vi "系统设置.vi"() -> ()   [LabVIEW 2016]
uses:
  <vilib>/Utility/miscctls.llb/LVPointTypeDef.ctl
  <vilib>/ptbypt/NI_PtbyPt.lvlib
  <vilib>/Utility/config.llb/NI_LVConfig.lvlib
  PLC/PLC.lvlib
panel:
  in  "模块启用配置":bool
  in  "短信报警设置":bool
  in  "首页显示设置":bool
  in  "跨度核查":bool
  in  "空白核查":bool
  out "选项卡控件":enum32{"自由设定", "国标协议", "流量设定"}(tab)
  in  "24H周期设置":bool[](xcontrol)
  in  "运行间隔":i16=4 min=1 max=24
  in  "流量阈值":dbl=4.0 min=1.0 max=24.0
  in  "时间阈值":u16=4 min=1 max=24
  in  "周期设置":enum16{"自由设定", "国标协议", "流量设定"}(ring)
  out "x = y?":bool
  in  "质控启动日期":string(combo)="关闭"
  in  "跨度核查时间":u16(ring)=6 items=["00H", "01H", "02H", "03H", "04H", "05H", "06H", "07H", "08H", "09H", "10H", "11H", "12H", "13H", "14H", "15H", "16H", "17H", "18H", "19H", "20H", "21H", "22H", "23H", "关闭"]
  in  "空白核查时间":u16(ring)=2 items=["00H", "01H", "02H", "03H", "04H", "05H", "06H", "07H", "08H", "09H", "10H", "11H", "12H", "13H", "14H", "15H", "16H", "17H", "18H", "19H", "20H", "21H", "22H", "23H", "关闭"]
  in  "CODCr":bool
  in  "总磷总氮":bool
  in  "氨氮":bool
  in  "CODmn":bool
  in  "多参数":bool
  in  "输入密码":dbl
  in  "布尔":bool
  in  "副屏显示设置":bool
  in  "开机启动":bool caption="氨氮禁用"
  in  "运行模式":enum16{"维护模式", "常规模式", "应急模式", "质控模式"}(ring)
  # "注：周期设置分为自由设定和国标协议两种。\n1：选择自由设定情况下：运行间隔将不可选用并变灰色，周期设置可自由手动勾选\n2：选择国标协议情况下：周期时间将由运行间隔选择的时间决定，下方周期设置被禁用并无法手动勾选。\n3：选择流量设定情况下：瞬时流量连续超过流量阈值到达时间阈值设定值，仪器将自动开启测量。"
  # "自动运行启动参数"
  # "质控频次："
  # "空白核查时间："
  # "跨度核查时间："
  # "启动周期设置"
  # "m3/S"
  # "秒"
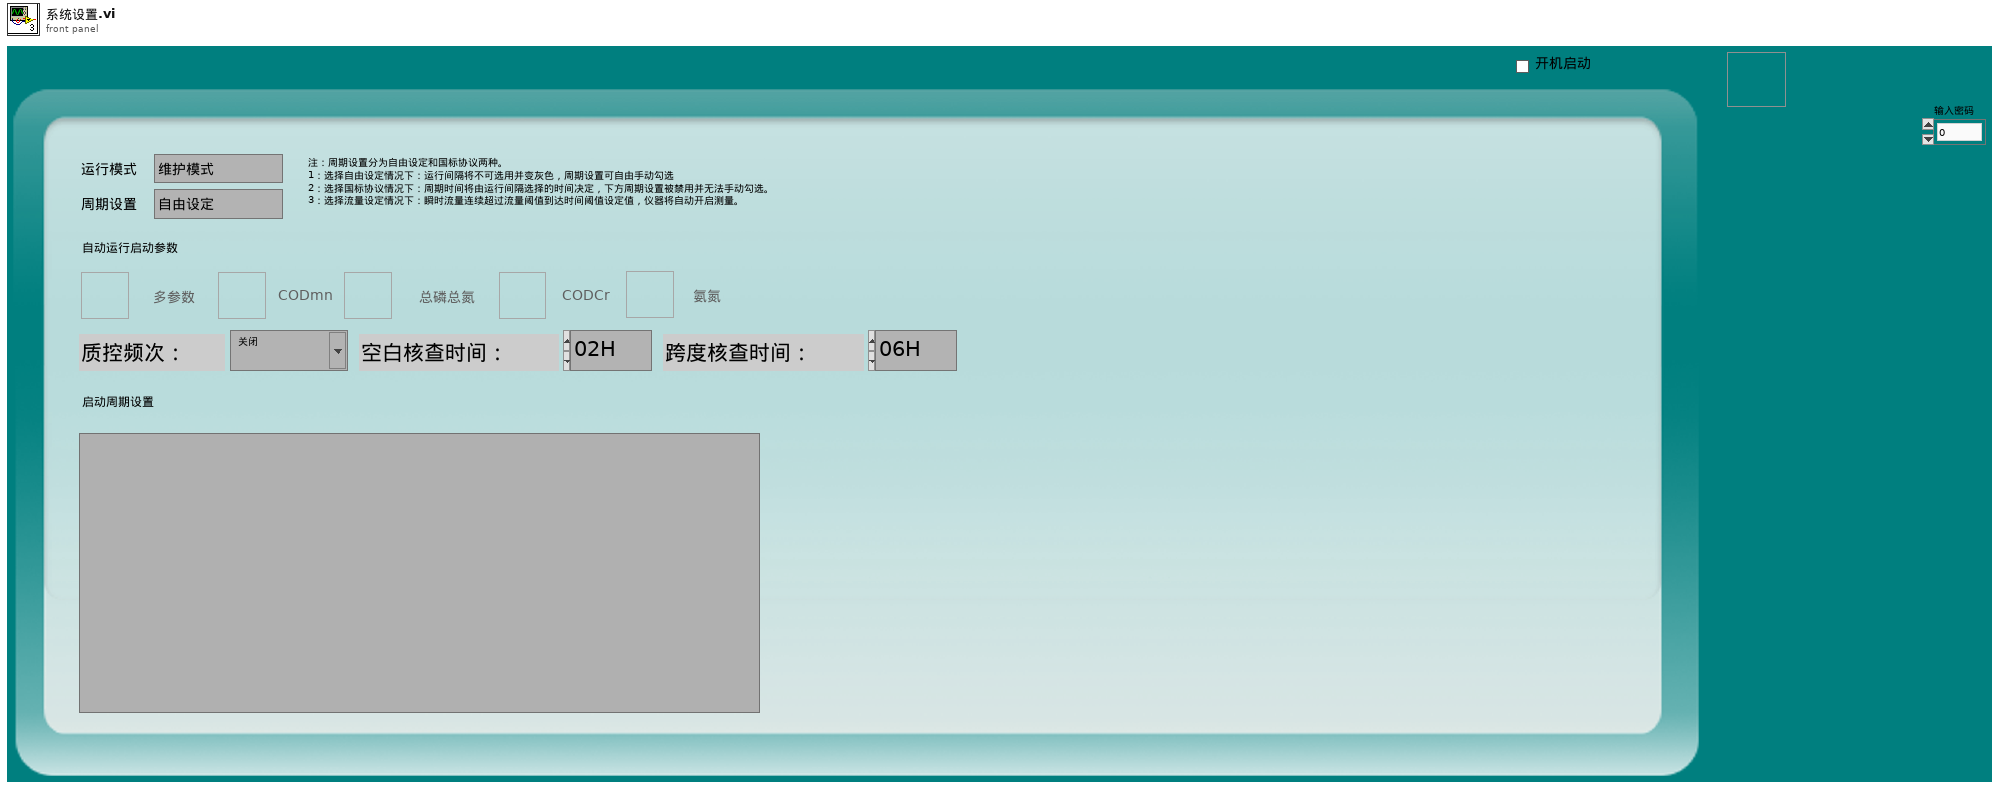
[diagram p1: front panel]
types:
  T1 = typedef "NI_LVConfig.lvlib/Config Data RefNum.ctl" = refnum<k1>
  T2 = typedef "LVPointTypeDef.ctl" = cluster{"Horizontal":i16, "Vertical":i16}
  T3 = enum8{"Enabled", "Disabled", "Disabled and Grayed Out"}
  T4 = enum32{"Bad", "Idle", "Run top level", "Running"}
  T5 = enum32{"Invalid", "Standard", "Closed", "Hidden", "Minimized", "Maximized"}
  T6 = cluster{"运行模式":enum16{"维护模式", "常规模式", "应急模式", "质控模式"}}
  T7 = cluster{"测量模式":enum16{"水样测量", "标样核查", "零点核查", "跨度核查", "空白测试", "加标回收", "平行样", "校零", "校标"}}
  T8 = cluster{"站号":u16, "量程切换":enum32{"H", "L", "AUTO"}, "控制命令":enum16{"启动测量", "标样核查", "零点核查", "跨度核查", "空白测试", "平行样测试", "加标回收", "空白校准", "标样校准", "初始化（清洗）", "停止测试", "仪器重启", "校时", "模式设置", "测量间隔设置"}, "模式设置":enum16{"待机", "连续模式", "周期模式", "定点模式", "受控模式", "手动模式"}, "测量间隔":u16}
  T9 = enum16{"启动测量", "标样核查", "零点核查", "跨度核查", "空白测试", "平行样测试", "加标回收", "空白校准", "标样校准", "初始化（清洗）", "停止测试", "仪器重启", "校时", "模式设置", "测量间隔设置"}
  T10 = cluster{"测试模式":enum16{"正常测试", "集成干预"}, "参数启用":cluster{"氨氮":bool, "总磷总氮":bool, "CODMn":bool, "CODcr":bool, "多参数":bool}}
  T11 = typedef "LVDateTimeRec.ctl" = cluster{"秒数的小数部分":dbl, "秒":i32, "分":i32, "时":i32, "日":i32, "月":i32, "年":i32, "天数（周）":i32, "天数（年）":i32, "DST":i32}
  T12 = cluster{"运行模式":enum16{"维护模式", "常规模式", "应急模式", "质控模式"}, "质控频次":enum16{"关闭", "每天", "星期一", "星期二", "星期三", "星期四", "星期五", "星期六", "星期日"}, "空白核查时间":u16, "跨度核查时间":u16, "24H周期设置":bool[]}
  T13 = cluster{"水样测试量程模式":enum16{"H", "L", "AUTO"}, "空白核查量程模式":enum16{"H", "L", "AUTO"}, "跨度核查量程模式":enum16{"H", "L", "AUTO"}}
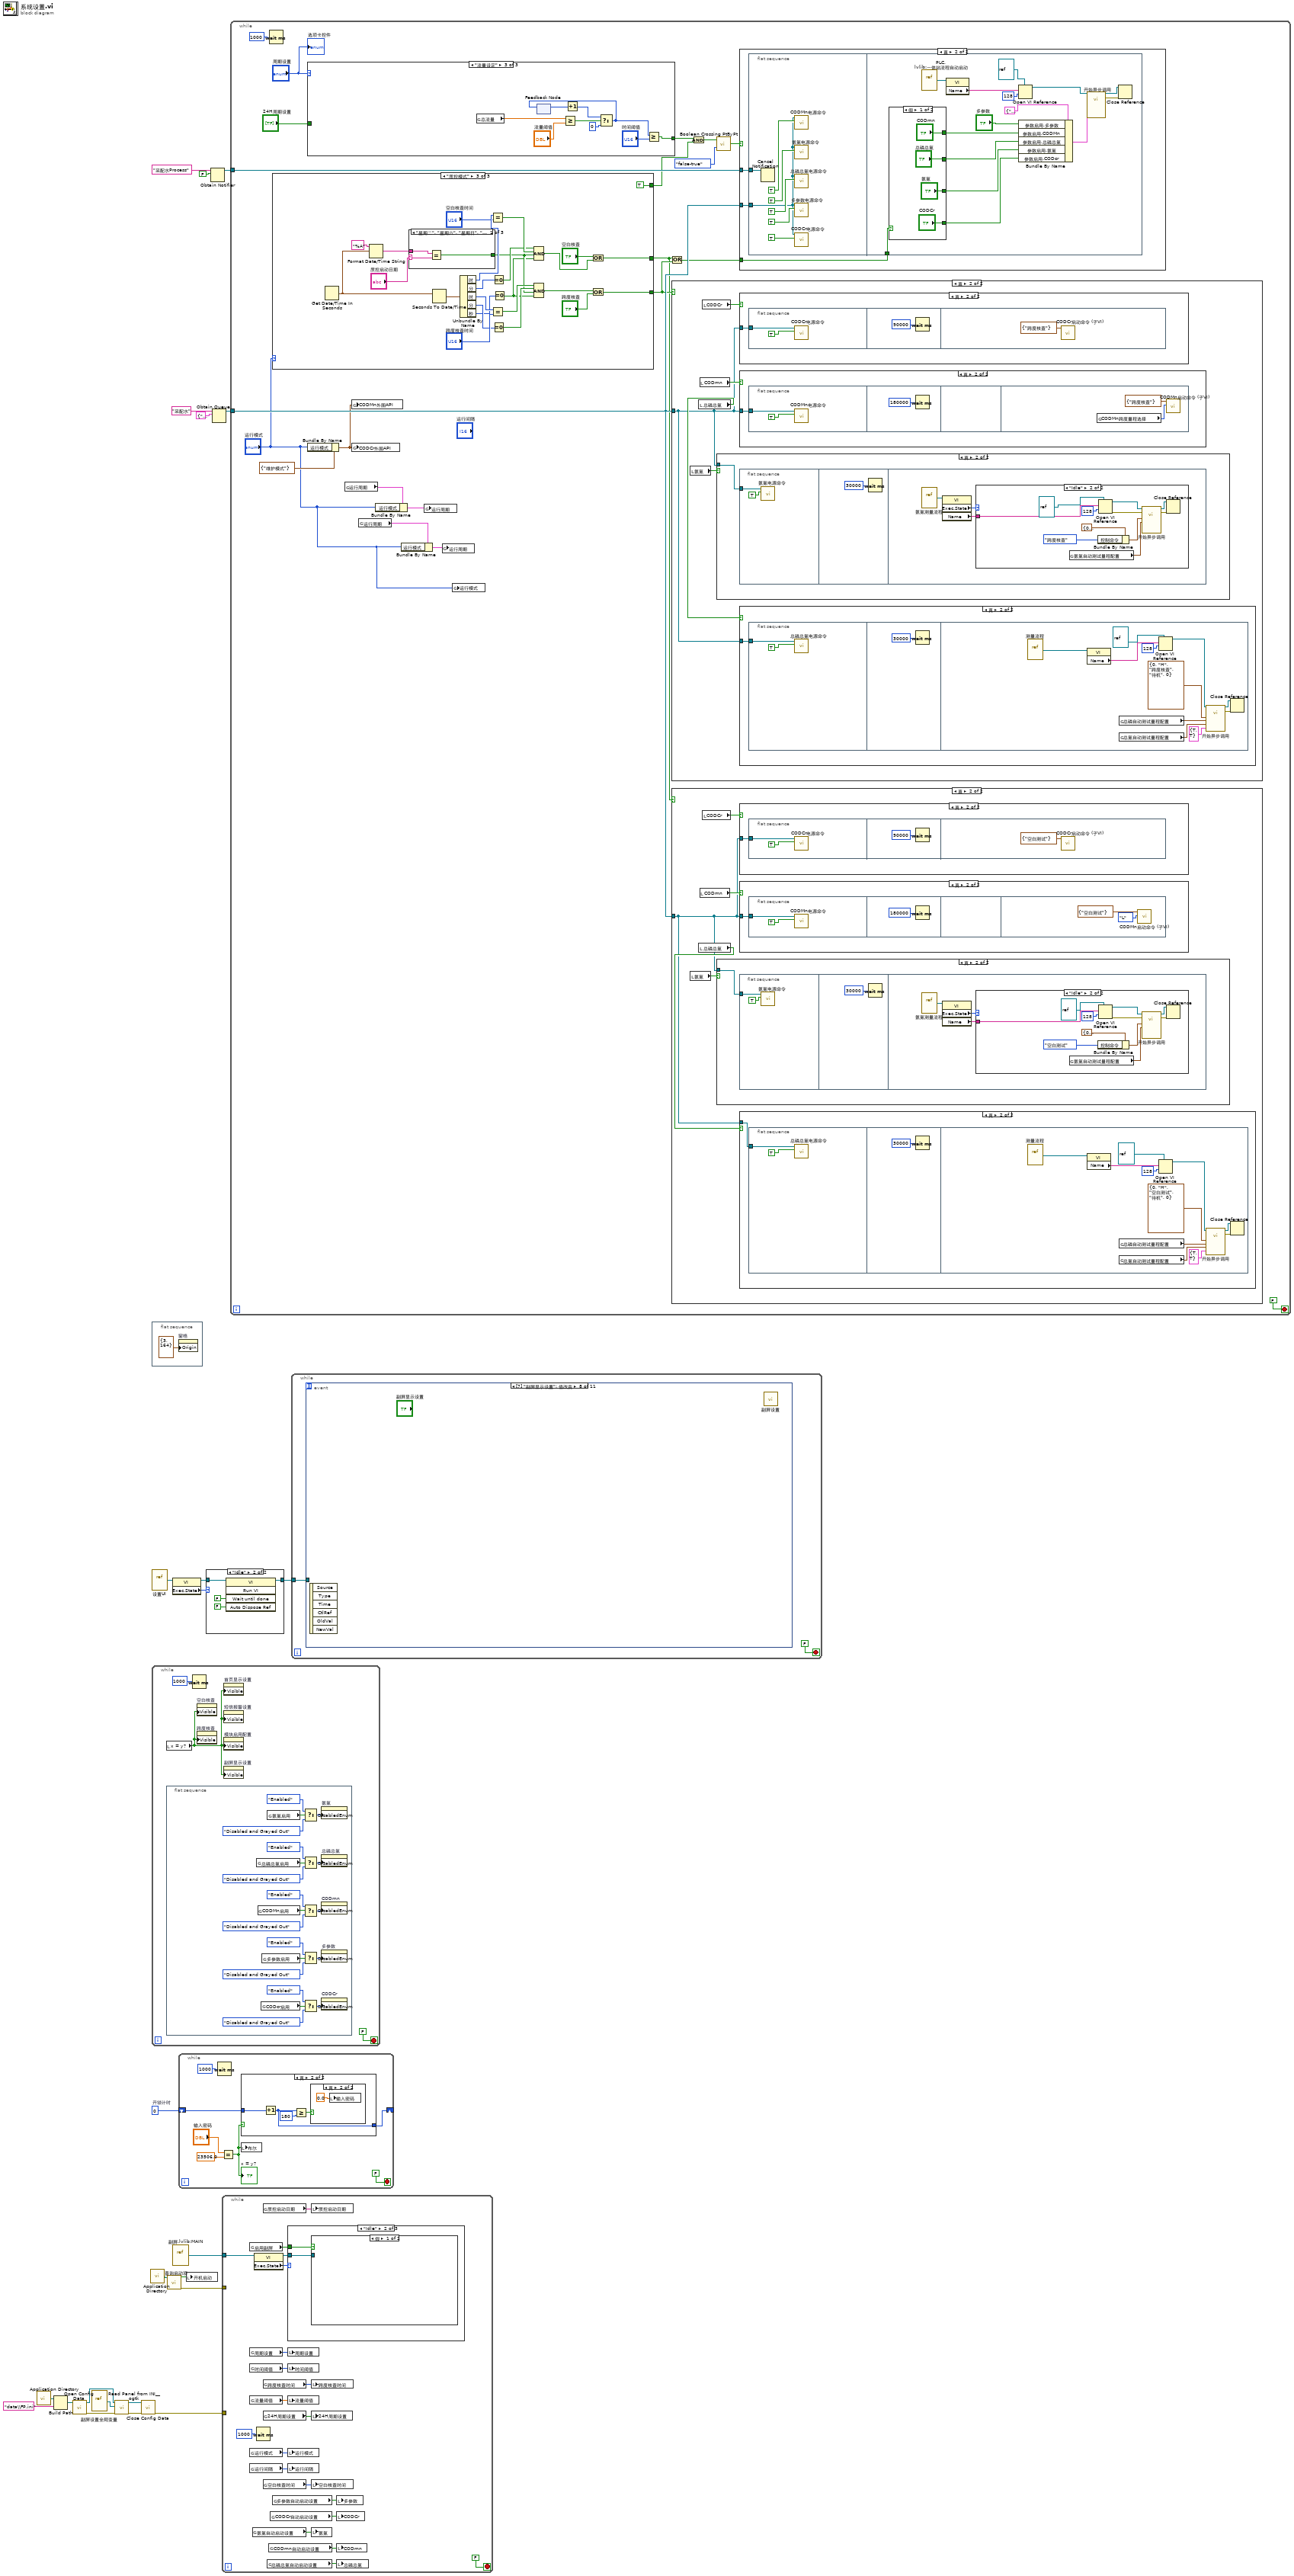
[diagram p0: block diagram]
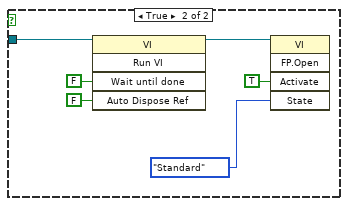
[diagram p6: hidden frame]
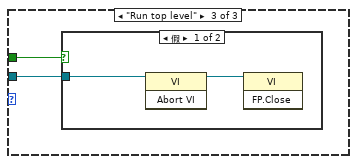
[diagram p7: hidden frame]
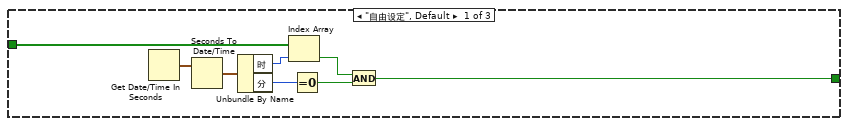
[diagram p9: hidden frame]
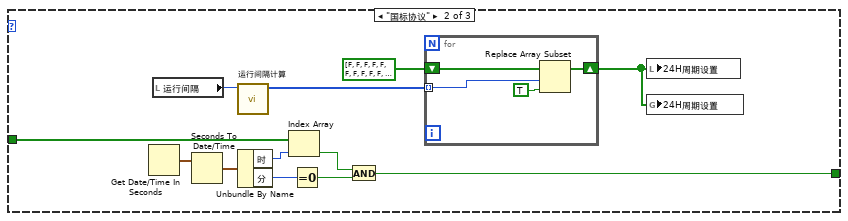
[diagram p10: hidden frame]
diagram:
  w19 = u32 0  # 开锁计时
  n1 = call <vilib>:"Application Directory.vi"() -> ("Application Directory"=w1:path)
  n2 = Build Path(base path=w1, name or relative path="data\\FP.ini" ("名称或相对路径")) -> (appended path=w8:path)
  n3 = call <vilib>:"Open Config Data.vi"("configuration file path"=w8) -> ("error out"=w7:errorcluster, "refnum"=w4:T1)  [unwired: 8 in, 1 out]
  n4 = vi-ref "副屏设置全局变量.vi"() -> (w5:refnum<vi>)
  n5 = call <userlib>:"Read Panel from INI__ogtk.vi"("error in (no error)"=w7, "VI ref"=w5, "refnum"=w4) -> ("error out"=w6:errorcluster, "refnum out"=w3:T1)  [unwired: 7 in]
  n6 = call <vilib>:"Close Config Data.vi"("error in (no error)"=w6, "refnum"=w3) -> ("error out"=w2:errorcluster)  [unwired: 8 in, 1 out]
  n7 = call <vilib>:"Application Directory.vi"() -> ("Application Directory"=w21:path)
  n8 = flat-sequence {
    frame #0 {
      n9 = property on="窗格" class="Pane"("Origin"=T2 {"Horizontal"=3, "Vertical"=164} ("原点")) -> ()  [unwired: 2 in, 2 out]
    }
  }
  n10 = vi-ref "设置UI.vi"() -> (w14:refnum<vi>)
  n11 = while {
    stop <- FALSE stop-if-true
    n12 = local read "x = y?"() -> (w26:bool)
    n13 = flat-sequence {
      frame #0 {
        n14 = global read "系统设置全局变量.vi" "总磷总氮启用"() -> (w36:bool)
        n15 = global read "系统设置全局变量.vi" "CODMn启用"() -> (w34:bool)
        n16 = global read "系统设置全局变量.vi" "CODcr启用"() -> (w35:bool)
        n17 = global read "系统设置全局变量.vi" "多参数启用"() -> (w33:bool)
        n18 = global read "系统设置全局变量.vi" "氨氮启用"() -> (w29:bool)
        n19 = Select(t=T3."Enabled" ("禁用"), s=w29, f=T3."Disabled and Grayed Out" ("禁用")) -> (s? t:f=w37:T3)
        n20 = Select(t=T3."Enabled" ("禁用"), s=w36, f=T3."Disabled and Grayed Out" ("禁用")) -> (s? t:f=w31:T3)
        n21 = Select(t=T3."Enabled" ("禁用"), s=w34, f=T3."Disabled and Grayed Out" ("禁用")) -> (s? t:f=w38:T3)
        n22 = Select(t=T3."Enabled" ("禁用"), s=w33, f=T3."Disabled and Grayed Out" ("禁用")) -> (s? t:f=w32:T3)
        n23 = Select(t=T3."Enabled" ("禁用"), s=w35, f=T3."Disabled and Grayed Out" ("禁用")) -> (s? t:f=w48:T3)
        n24 = property on="氨氮" class="Bool (严格)"("DisabledEnum"=w37) -> ()  [unwired: 2 in, 2 out]
        n25 = property on="总磷总氮" class="Bool (严格)"("DisabledEnum"=w31) -> ()  [unwired: 2 in, 2 out]
        n26 = property on="CODmn" class="Bool (严格)"("DisabledEnum"=w38) -> ()  [unwired: 2 in, 2 out]
        n27 = property on="多参数" class="Bool (严格)"("DisabledEnum"=w32) -> ()  [unwired: 2 in, 2 out]
        n28 = property on="CODCr" class="Bool (严格)"("DisabledEnum"=w48) -> ()  [unwired: 2 in, 2 out]
      }
    }
    n29 = Wait (ms)(milliseconds to wait=u32 1000 ("等待时间（毫秒）")) -> ()  [unwired: 1 out]
    n30 = property on="空白核查" class="Bool"("Visible"=w26) -> ()  [unwired: 2 in, 2 out]
    n31 = property on="跨度核查" class="Bool"("Visible"=w26) -> ()  [unwired: 2 in, 2 out]
    n32 = property on="首页显示设置" class="Bool"("Visible"=w26) -> ()  [unwired: 2 in, 2 out]
    n33 = property on="短信报警设置" class="Bool"("Visible"=w26) -> ()  [unwired: 2 in, 2 out]
    n34 = property on="模块启用配置" class="Bool"("Visible"=w26) -> ()  [unwired: 2 in, 2 out]
    n35 = property on="副屏显示设置" class="Bool"("Visible"=w26) -> ()  [unwired: 2 in, 2 out]
  }
  n36 = call "查询启动项.vi"("启动文件路径"=w21) -> ("error out"=w10:errorcluster, "包含启动项"=w20:bool)  [unwired: 9 in]
  n37 = property class="VI"(reference=w14) -> (reference out=w12:refnum<vi>, "Exec.State"=w13:T4)  [unwired: 1 in, 1 out]
  n38 = vi-ref "副屏.lvlib:MAIN.vi"() -> (w15:refnum<vi>)
  n39 = while {
    shift-right: [w50] -> _
    shift-left: w19 -> [w51]
    stop <- FALSE stop-if-true
    n40 = Wait (ms)(milliseconds to wait=u32 1000 ("等待时间（毫秒）")) -> ()  [unwired: 1 out]
    n41 = Equal?(x="输入密码", y=23506.0) -> (x = y?=w49:bool)
    "x = y?" <- w49
    n42 = case shown="真" w49 {
      tunnel: w51 -> [_ w59]
      tunnel: [_ w58] -> w50
      frame False {
      }
      frame True {
        n43 = Increment(x=w59) -> (x+1=w58:u32)
        n44 = Greater Or Equal?(x=w58, y=u32 180) -> (x >= y?=w56:bool)
        n45 = case shown="真" w56 {
          frame False {
          }
          frame True {
            n46 = local write "输入密码"(0.0 ("输入密码")) -> ()
          }
        }
      }
    }
    n47 = local write "布尔"(w49) -> ()
  }
  n48 = local write "开机启动"(w20) -> ()
  n49 = case shown="\"Idle\"" w13 {
    tunnel: w12 -> [w61 w65]
    tunnel: [w61 w64] -> w11
    frame "Bad", Default {
    }
    frame "Idle" {
      n50 = invoke class="VI" method="Run VI"(reference=w65, "Wait until done"=FALSE ("结束前等待"), "Auto Dispose Ref"=FALSE ("自动销毁引用")) -> (reference out=w64:refnum<vi>)  [unwired: 2 in, 4 out]
    }
  }
  n51 = Obtain Notifier(name (unnamed)="采配水Process" ("名称（未命名）"), notification data type=FALSE) -> (notifier out=w22:refnum<notifier>)  [unwired: 2 in, 2 out]
  n52 = Obtain Queue(name (unnamed)="采配水" ("名称（未命名）"), element data type=cluster{"命令":string, "数据":variant} {"命令"="", "数据"=variant}) -> (queue out=w16:refnum<queue>)  [unwired: 3 in, 2 out]
  n53 = while {
    tunnel: w15 -> [w77]
    tunnel: w10 -> [_]
    tunnel: w2 -> [_]
    stop <- FALSE stop-if-true
    n54 = global read "副屏设置全局变量.vi" "启用副屏"() -> (w75:bool)
    n55 = global read "系统设置全局变量.vi" "周期设置"() -> (w70:enum16{"自由设定", "国标协议", "流量设定"})
    n56 = global read "系统设置全局变量.vi" "时间阈值"() -> (w66:u16)
    n57 = global read "系统设置全局变量.vi" "流量阈值"() -> (w67:dbl)
    n58 = global read "系统设置全局变量.vi" "运行模式"() -> (w68:enum16{"维护模式", "常规模式", "应急模式", "质控模式"})
    n59 = global read "系统设置全局变量.vi" "运行间隔"() -> (w69:i16)
    n60 = global read "系统设置全局变量.vi" "氨氮自动启动设置"() -> (w82:bool)
    n61 = property class="VI"(reference=w77) -> (reference out=w74:refnum<vi>, "Exec.State"=w76:T4)  [unwired: 1 in, 1 out]
    n62 = Wait (ms)(milliseconds to wait=u32 1000 ("等待时间（毫秒）")) -> ()  [unwired: 1 out]
    n63 = global read "系统设置全局变量.vi" "质控启动日期"() -> (w73:string)
    n64 = global read "系统设置全局变量.vi" "跨度核查时间"() -> (w71:u16)
    n65 = global read "系统设置全局变量.vi" "24H周期设置"() -> (w83:bool[])
    n66 = global read "系统设置全局变量.vi" "空白核查时间"() -> (w72:u16)
    n67 = global read "系统设置全局变量.vi" "总磷总氮自动启动设置"() -> (w80:bool)
    n68 = global read "系统设置全局变量.vi" "CODmn自动启动设置"() -> (w79:bool)
    n69 = global read "系统设置全局变量.vi" "CODCr自动启动设置"() -> (w81:bool)
    n70 = global read "系统设置全局变量.vi" "多参数自动启动设置"() -> (w78:bool)
    n71 = case shown="\"Idle\"" w76 {
      tunnel: w75 -> [_ w86 w94]
      tunnel: w74 -> [_ w87 w95]
      frame "Bad", Default {
      }
      frame "Idle" {
        n72 = case shown="假" w86 {
          tunnel: w87 -> [_ w93]
          frame False {
          }
          frame True {
            n73 = invoke class="VI" method="Run VI"(reference=w93, "Wait until done"=FALSE ("结束前等待"), "Auto Dispose Ref"=FALSE ("自动销毁引用")) -> (reference out=w88:refnum<vi>)  [unwired: 2 in, 4 out]
            n74 = invoke class="VI" method="FP.Open"(reference=w88, "Activate"=TRUE ("激活？"), "State"=T5."Standard" ("状态")) -> ()  [unwired: 2 in, 5 out]
          }
        }
      }
      frame "Run top level" {
        n75 = case shown="假" w94 {
          tunnel: w95 -> [w96 _]
          frame False {
            n76 = invoke class="VI" method="Abort VI"(reference=w96) -> (reference out=w97:refnum<vi>)  [unwired: 2 in, 2 out]
            n77 = invoke class="VI" method="FP.Close"(reference=w97) -> ()  [unwired: 2 in, 3 out]
          }
          frame True {
          }
        }
      }
    }
    n78 = local write "周期设置"(w70) -> ()
    n79 = local write "时间阈值"(w66) -> ()
    n80 = local write "流量阈值"(w67) -> ()
    n81 = local write "运行模式"(w68) -> ()
    n82 = local write "运行间隔"(w69) -> ()
    n83 = local write "质控启动日期"(w73) -> ()
    n84 = local write "跨度核查时间"(w71) -> ()
    n85 = local write "24H周期设置"(w83) -> ()
    n86 = local write "空白核查时间"(w72) -> ()
    n87 = local write "氨氮"(w82) -> ()
    n88 = local write "多参数"(w78) -> ()
    n89 = local write "CODCr"(w81) -> ()
    n90 = local write "CODmn"(w79) -> ()
    n91 = local write "总磷总氮"(w80) -> ()
  }
  n92 = while {
    tunnel: w22 -> [w116]
    tunnel: w16 -> [w112]
    stop <- FALSE stop-if-true
    n93 = Wait (ms)(milliseconds to wait=u32 1000 ("等待时间（毫秒）")) -> ()  [unwired: 1 out]
    n94 = case shown="\"质控模式\"" "运行模式" {
      tunnel: [_ _ w280] -> w106
      tunnel: [_ _ w284] -> w105
      tunnel: [_ TRUE TRUE] -> w109
      frame "维护模式", Default {
      }
      frame "常规模式" {
      }
      frame "质控模式" {
        n95 = Get Date/Time In Seconds() -> (seconds since 1Jan1904=w291:timestamp)
        n96 = Format Date/Time String(time format string (%c)="%A" ("时间格式字符串(%c)"), seconds (now)=w291) -> (date/time string=w289:string)  [unwired: 1 in]
        n97 = case shown="\"星期二\", \"星期六\", \"星期日\", \"星期三\", \"星期四\", \"星期五\", \"星期一\"" "质控启动日期" {
          selector: "质控启动日期" -> [w307 _ _]
          tunnel: [w306 TRUE FALSE] -> w292
          tunnel: w289 -> [w305 _ _]
          frame "星期二", "星期六", "星期日", "星期三", "星期四", "星期五", "星期一" {
            n98 = Equal?(x=w305, y=w307) -> (x = y?=w306:bool)
          }
          frame "每天" {
          }
          frame "关闭", Default {
          }
        }
        n99 = Seconds To Date/Time(time stamp (now)=w291) -> (date time rec=w304:T11)  [unwired: 1 in]
        n100 = Unbundle By Name(w304) -> ("时"=w303:i32, "分"=w301:i32, "时"=w297:i32, "分"=w296:i32, "秒"=w288:i32)
        n101 = Equal?(x=w303, y="空白核查时间") -> (x = y?=w300:bool)
        n102 = Equal?(x=w297, y="跨度核查时间") -> (x = y?=w295:bool)
        n103 = Equal To 0?(x=w301) -> (x = 0?=w299:bool)
        n104 = Equal To 0?(x=w296) -> (x = 0?=w294:bool)
        n105 = Equal To 0?(x=w288) -> (x = 0?=w287:bool)
        n106 = Compound Arithmetic op=AND ("复合运算")(w299, w300, w292, w287) -> (w285:bool)
        n107 = Compound Arithmetic op=AND ("复合运算")(w295, w294, w292, w287) -> (w282:bool)
        n108 = Or(x="空白核查", y=w285) -> (x .or. y?=w284:bool)
        n109 = Or(x=w282, y="跨度核查") -> (x .or. y?=w280:bool)
      }
    }
    n110 = case shown="\"流量设定\"" "周期设置" {
      tunnel: [w120 w127 w143] -> w108
      tunnel: "24H周期设置" -> [w119 w128 _]
      frame "自由设定", Default {
        n111 = Get Date/Time In Seconds() -> (seconds since 1Jan1904=w121:timestamp)
        n112 = Seconds To Date/Time(time stamp (now)=w121) -> (date time rec=w122:T11)  [unwired: 1 in]
        n113 = Unbundle By Name(w122) -> ("时"=w125:i32, "分"=w123:i32)
        n114 = Index Array(array=w119, index=w125) -> (element=w126:bool)
        n115 = Equal To 0?(x=w123) -> (x = 0?=w124:bool)
        n116 = And(x=w126, y=w124) -> (x .and. y?=w120:bool)
      }
      frame "国标协议" {
        n117 = Get Date/Time In Seconds() -> (seconds since 1Jan1904=w129:timestamp)
        n118 = local read "运行间隔"() -> (w138:i16)
        n119 = Seconds To Date/Time(time stamp (now)=w129) -> (date time rec=w130:T11)  [unwired: 1 in]
        n120 = call "运行间隔计算.vi"("运行周期"=w138) -> ("数组"=w137:i32[])  [unwired: 10 in]
        n121 = Unbundle By Name(w130) -> ("时"=w133:i32, "分"=w131:i32)
        n122 = Index Array(array=w128, index=w133) -> (element=w134:bool)
        n123 = Equal To 0?(x=w131) -> (x = 0?=w132:bool)
        n124 = And(x=w134, y=w132) -> (x .and. y?=w127:bool)
        n125 = for {
          tunnel: w137 -> [w141] mode=indexing
          shift-right: [w139] -> w135
          shift-left: bool[] [FALSE, FALSE, FALSE, FALSE, FALSE, FALSE, FALSE, FALSE, FALSE, FALSE, FALSE, FALSE, FALSE, FALSE, FALSE, FALSE, FALSE, FALSE, FALSE, FALSE, FALSE, FALSE, FALSE, FALSE] ("24H周期设置") -> [w142]
          n126 = Replace Array Subset(array=w142, new element=TRUE ("新元素/子数组"), index=w141) -> (w139:bool[])
        }
        n127 = local write "24H周期设置"(w135) -> ()
        n128 = global write "系统设置全局变量.vi" "24H周期设置"(w135) -> ()
      }
      frame "流量设定" {
        n129 = global read "流量计全局变量.vi" "总流量"() -> (w151:dbl)
        n130 = feedback #1() -> (w148:i16)  [unwired: 1 in]
        n131 = Greater Or Equal?(x=w151, y="流量阈值") -> (x >= y?=w146:bool)
        n132 = Increment(x=w148) -> (x+1=w147:i16)
        n133 = Select(t=w147, s=w146, f=i16 0) -> (s? t:f=w145:i16)
        n134 = feedback-in #1(w145) -> ()
        n135 = Greater Or Equal?(x=w145, y="时间阈值") -> (x >= y?=w143:bool)
      }
    }
    n136 = Bundle By Name(cluster=T6 {"运行模式"=enum."维护模式"} ("外围API"), "运行模式"="运行模式") -> (w103:T6)
    n137 = global read "总磷总氮断电保存全局变量.vi" "运行周期"() -> (w102:T12)
    n138 = global write "CODMN外部API.vi" "CODMn外围API"(w103) -> ()
    n139 = global write "CODCr外部API.vi" "CODCr外围API"(w103) -> ()
    n140 = global read "氨氮断电保存全局变量.vi" "运行周期"() -> (w100:T12)
    n141 = Bundle By Name(cluster=w102, "运行模式"="运行模式") -> (w101:T12)
    n142 = Bundle By Name(cluster=w100, "运行模式"="运行模式") -> (w99:T12)
    n143 = global write "总磷总氮断电保存全局变量.vi" "运行周期"(w101) -> ()
    n144 = global write "氨氮断电保存全局变量.vi" "运行周期"(w99) -> ()
    n145 = global write "多参数全局变量.vi" "运行模式"("运行模式") -> ()
    n146 = Or(x=w105, y=w106) -> (x .or. y?=w104:bool)
    n147 = case shown="真" w106 {
      tunnel: w112 -> [_ w152]
      frame False {
      }
      frame True {
        n148 = local read "氨氮"() -> (w156:bool)
        n149 = local read "总磷总氮"() -> (w155:bool)
        n150 = local read "CODmn"() -> (w154:bool)
        n151 = local read "CODCr"() -> (w153:bool)
        n152 = case shown="真" w156 {
          tunnel: w152 -> [_ w183]
          frame False {
          }
          frame True {
            n153 = flat-sequence {
              tunnel: w183 -> [w184]
              frame #0 {
                n154 = call "氨氮电源命令.vi"("通电/断电"=TRUE, "队列"=w184) -> ()  [unwired: 9 in, 1 out]
              }
              frame #1 {
                n155 = Wait (ms)(milliseconds to wait=u32 30000 ("等待时间（毫秒）")) -> ()  [unwired: 1 out]
              }
              frame #2 {
                n156 = vi-ref "氨氮测量流程.vi"() -> (w189:refnum<vi>)
                n157 = property class="VI"(reference=w189) -> ("Exec.State"=w187:T4, "Name"=w188:string)  [unwired: 1 in, 2 out]
                n158 = case shown="\"Idle\"" w187 {
                  tunnel: w188 -> [_ w197]
                  frame "Bad", Default {
                  }
                  frame "Idle" {
                    n159 = global read "氨氮断电保存全局变量.vi" "氨氮自动测试量程配置"() -> (w191:T13)
                    n160 = Bundle By Name(cluster=T8 {"站号"=0, "量程切换"=enum."H", "控制命令"=enum."启动测量", "模式设置"=enum."待机", "测量间隔"=0} ("参数"), "控制命令"=T9."跨度核查") -> (w192:T8)
                    n161 = Open VI Reference(type specifier VI Refnum (for type only)=refnum<vi> refnum, vi path=w197, options=128 ("选项")) -> (vi reference=w193:refnum<vi>, error out=w198:errorcluster)  [unwired: 3 in]
                    n162 = call-by-ref "开始异步调用"(reference=w193, error in=w198, "量程模式"=w191, "参数"=w192) -> (reference out=w199:refnum<vi>, error out=w200:errorcluster)  [unwired: 10 in]
                    n163 = Close Reference(reference=w199, error in (no error)=w200) -> ()  [unwired: 1 out]
                  }
                }
              }
            }
          }
        }
        n164 = case shown="真" w153 {
          tunnel: w152 -> [_ w157]
          frame False {
          }
          frame True {
            n165 = flat-sequence {
              tunnel: w157 -> [w158]
              frame #0 {
                n166 = call "CODCr电源命令.vi"("通电/断电"=TRUE, "队列"=w158) -> ()  [unwired: 9 in, 1 out]
              }
              frame #1 {
                n167 = Wait (ms)(milliseconds to wait=u32 90000 ("等待时间（毫秒）")) -> ()  [unwired: 1 out]
              }
              frame #2 {
                n168 = call "CODCr启动命令 (子VI).vi"("启动测量模式"=T7 {"测量模式"=enum."跨度核查"}) -> ()  [unwired: 11 in]
              }
            }
          }
        }
        n169 = case shown="真" w154 {
          tunnel: w152 -> [_ w162]
          frame False {
          }
          frame True {
            n170 = flat-sequence {
              tunnel: w162 -> [w163]
              frame #0 {
                n171 = call "CODMn电源命令.vi"("通电/断电"=TRUE, "队列"=w163) -> ()  [unwired: 9 in, 1 out]
              }
              frame #1 {
                n172 = Wait (ms)(milliseconds to wait=u32 180000 ("等待时间（毫秒）")) -> ()  [unwired: 1 out]
              }
              frame #2 {
              }
              frame #3 {
                n173 = global read "CODMn断电保存全局变量.vi" "CODMn跨度量程选择"() -> (w166:enum32{"H", "L", "AUTO"})
                n174 = call "CODMn启动命令 (子VI).vi"("CODMn量程切换"=w166, "启动测量模式"=T7 {"测量模式"=enum."跨度核查"}) -> ()  [unwired: 10 in]
              }
            }
          }
        }
        n175 = case shown="真" w155 {
          tunnel: w152 -> [_ w168]
          frame False {
          }
          frame True {
            n176 = flat-sequence {
              tunnel: w168 -> [w170]
              frame #0 {
                n177 = call "总磷总氮电源命令.vi"("通电/断电"=TRUE, "队列"=w170) -> ()  [unwired: 9 in, 1 out]
              }
              frame #1 {
                n178 = Wait (ms)(milliseconds to wait=u32 30000 ("等待时间（毫秒）")) -> ()  [unwired: 1 out]
              }
              frame #2 {
                n179 = vi-ref "测量流程.vi"() -> (w180:refnum<vi>)
                n180 = property class="VI"(reference=w180) -> ("Name"=w181:string)  [unwired: 1 in, 2 out]
                n181 = global read "总磷总氮断电保存全局变量.vi" "总磷自动测试量程配置"() -> (w175:T13)
                n182 = global read "总磷总氮断电保存全局变量.vi" "总氮自动测试量程配置"() -> (w174:T13)
                n183 = Open VI Reference(type specifier VI Refnum (for type only)=refnum<vi> refnum, vi path=w181, options=128 ("选项")) -> (vi reference=w179:refnum<vi>)  [unwired: 3 in, 1 out]
                n184 = call-by-ref "开始异步调用"(reference=w179, "启动参数"=cluster{"总磷":bool, "总氮":bool} {"总磷"=TRUE, "总氮"=TRUE}, "总氮量程模式"=w174, "总磷量程模式"=w175, "参数"=T8 {"站号"=0, "量程切换"=enum."H", "控制命令"=enum."跨度核查", "模式设置"=enum."待机", "测量间隔"=0}) -> (reference out=w178:refnum<vi>, error out=w177:errorcluster)  [unwired: 9 in]
                n185 = Close Reference(reference=w178, error in (no error)=w177) -> ()  [unwired: 1 out]
              }
            }
          }
        }
      }
    }
    n186 = case shown="真" w105 {
      tunnel: w112 -> [_ w201]
      frame False {
      }
      frame True {
        n187 = local read "氨氮"() -> (w205:bool)
        n188 = local read "总磷总氮"() -> (w204:bool)
        n189 = local read "CODmn"() -> (w203:bool)
        n190 = local read "CODCr"() -> (w202:bool)
        n191 = case shown="真" w205 {
          tunnel: w201 -> [_ w232]
          frame False {
          }
          frame True {
            n192 = flat-sequence {
              tunnel: w232 -> [w233]
              frame #0 {
                n193 = call "氨氮电源命令.vi"("通电/断电"=TRUE, "队列"=w233) -> ()  [unwired: 9 in, 1 out]
              }
              frame #1 {
                n194 = Wait (ms)(milliseconds to wait=u32 30000 ("等待时间（毫秒）")) -> ()  [unwired: 1 out]
              }
              frame #2 {
                n195 = vi-ref "氨氮测量流程.vi"() -> (w238:refnum<vi>)
                n196 = property class="VI"(reference=w238) -> ("Exec.State"=w236:T4, "Name"=w237:string)  [unwired: 1 in, 2 out]
                n197 = case shown="\"Idle\"" w236 {
                  tunnel: w237 -> [_ w246]
                  frame "Bad", Default {
                  }
                  frame "Idle" {
                    n198 = global read "氨氮断电保存全局变量.vi" "氨氮自动测试量程配置"() -> (w239:T13)
                    n199 = Bundle By Name(cluster=T8 {"站号"=0, "量程切换"=enum."H", "控制命令"=enum."启动测量", "模式设置"=enum."待机", "测量间隔"=0} ("参数"), "控制命令"=T9."空白测试") -> (w241:T8)
                    n200 = Open VI Reference(type specifier VI Refnum (for type only)=refnum<vi> refnum, vi path=w246, options=128 ("选项")) -> (vi reference=w242:refnum<vi>, error out=w247:errorcluster)  [unwired: 3 in]
                    n201 = call-by-ref "开始异步调用"(reference=w242, error in=w247, "量程模式"=w239, "参数"=w241) -> (reference out=w248:refnum<vi>, error out=w249:errorcluster)  [unwired: 10 in]
                    n202 = Close Reference(reference=w248, error in (no error)=w249) -> ()  [unwired: 1 out]
                  }
                }
              }
            }
          }
        }
        n203 = case shown="真" w202 {
          tunnel: w201 -> [_ w206]
          frame False {
          }
          frame True {
            n204 = flat-sequence {
              tunnel: w206 -> [w207]
              frame #0 {
                n205 = call "CODCr电源命令.vi"("通电/断电"=TRUE, "队列"=w207) -> ()  [unwired: 9 in, 1 out]
              }
              frame #1 {
                n206 = Wait (ms)(milliseconds to wait=u32 90000 ("等待时间（毫秒）")) -> ()  [unwired: 1 out]
              }
              frame #2 {
                n207 = call "CODCr启动命令 (子VI).vi"("启动测量模式"=T7 {"测量模式"=enum."空白测试"}) -> ()  [unwired: 11 in]
              }
            }
          }
        }
        n208 = case shown="真" w203 {
          tunnel: w201 -> [_ w211]
          frame False {
          }
          frame True {
            n209 = flat-sequence {
              tunnel: w211 -> [w212]
              frame #0 {
                n210 = call "CODMn电源命令.vi"("通电/断电"=TRUE, "队列"=w212) -> ()  [unwired: 9 in, 1 out]
              }
              frame #1 {
                n211 = Wait (ms)(milliseconds to wait=u32 180000 ("等待时间（毫秒）")) -> ()  [unwired: 1 out]
              }
              frame #2 {
              }
              frame #3 {
                n212 = call "CODMn启动命令 (子VI).vi"("CODMn量程切换"=enum32{"H", "L", "AUTO"}."L", "启动测量模式"=T7 {"测量模式"=enum."空白测试"}) -> ()  [unwired: 10 in]
              }
            }
          }
        }
        n213 = case shown="真" w204 {
          tunnel: w201 -> [_ w217]
          frame False {
          }
          frame True {
            n214 = flat-sequence {
              tunnel: w217 -> [w219]
              frame #0 {
                n215 = call "总磷总氮电源命令.vi"("通电/断电"=TRUE, "队列"=w219) -> ()  [unwired: 9 in, 1 out]
              }
              frame #1 {
                n216 = Wait (ms)(milliseconds to wait=u32 30000 ("等待时间（毫秒）")) -> ()  [unwired: 1 out]
              }
              frame #2 {
                n217 = vi-ref "测量流程.vi"() -> (w229:refnum<vi>)
                n218 = property class="VI"(reference=w229) -> ("Name"=w230:string)  [unwired: 1 in, 2 out]
                n219 = global read "总磷总氮断电保存全局变量.vi" "总磷自动测试量程配置"() -> (w223:T13)
                n220 = global read "总磷总氮断电保存全局变量.vi" "总氮自动测试量程配置"() -> (w222:T13)
                n221 = Open VI Reference(type specifier VI Refnum (for type only)=refnum<vi> refnum, vi path=w230, options=128 ("选项")) -> (vi reference=w228:refnum<vi>)  [unwired: 3 in, 1 out]
                n222 = call-by-ref "开始异步调用"(reference=w228, "启动参数"=cluster{"总磷":bool, "总氮":bool} {"总磷"=TRUE, "总氮"=TRUE}, "总氮量程模式"=w222, "总磷量程模式"=w223, "参数"=T8 {"站号"=0, "量程切换"=enum."H", "控制命令"=enum."空白测试", "模式设置"=enum."待机", "测量间隔"=0}) -> (reference out=w227:refnum<vi>, error out=w226:errorcluster)  [unwired: 9 in]
                n223 = Close Reference(reference=w227, error in (no error)=w226) -> ()  [unwired: 1 out]
              }
            }
          }
        }
      }
    }
    n224 = And(x=w108, y=w109) -> (x .and. y?=w107:bool)
    n225 = call <vilib>:"Boolean Crossing PtByPt.vi"("direction"=enum16{"either", "false-true", "true-false"}."false-true", "input"=w107) -> ("crossing"=w114:bool)  [unwired: 1 in]
    n226 = case shown="真" w114 {
      tunnel: w116 -> [_ w252]
      tunnel: w112 -> [_ w251]
      tunnel: w104 -> [_ w250]
      frame False {
      }
      frame True {
        n227 = flat-sequence {
          tunnel: w252 -> [w259]
          tunnel: w251 -> [w253]
          tunnel: w250 -> [w263]
          frame #0 {
            n228 = Cancel Notification(0:w259) -> ()  [unwired: 1 in, 3 out]
            n229 = call "CODMn电源命令.vi"("通电/断电"=TRUE, "队列"=w253) -> ()  [unwired: 9 in, 1 out]
            n230 = call "氨氮电源命令.vi"("通电/断电"=TRUE, "队列"=w253) -> ()  [unwired: 9 in, 1 out]
            n231 = call "总磷总氮电源命令.vi"("通电/断电"=TRUE, "队列"=w253) -> ()  [unwired: 9 in, 1 out]
            n232 = call "多参数电源命令.vi"("通电/断电"=TRUE, "队列"=w253) -> ()  [unwired: 9 in, 1 out]
            n233 = call "CODCr电源命令.vi"("通电/断电"=TRUE, "队列"=w253) -> ()  [unwired: 9 in, 1 out]
          }
          frame #1 {
            n234 = case shown="假" w263 {
              tunnel: ["CODmn" _] -> w273
              tunnel: ["总磷总氮" _] -> w272
              tunnel: ["CODCr" _] -> w271
              tunnel: ["氨氮" _] -> w270
              frame False {
              }
              frame True {
              }
            }
            n235 = vi-ref "PLC.lvlib:一体站流程自动启动.vi"() -> (w267:refnum<vi>)
            n236 = property class="VI"(reference=w267) -> ("Name"=w268:string)  [unwired: 1 in, 2 out]
            n237 = Bundle By Name(cluster=T10 {"测试模式"=enum."正常测试", "参数启用"={"氨氮"=FALSE, "总磷总氮"=FALSE, "CODMn"=FALSE, "CODcr"=FALSE, "多参数"=FALSE}} ("参数"), "参数启用.多参数"="多参数", "参数启用.CODMn"=w273, "参数启用.总磷总氮"=w272, "参数启用.氨氮"=w270, "参数启用.CODcr"=w271) -> (w260:T10)
            n238 = Open VI Reference(type specifier VI Refnum (for type only)=refnum<vi> refnum, vi path=w268, options=128 ("选项")) -> (vi reference=w266:refnum<vi>)  [unwired: 3 in, 1 out]
            n239 = call-by-ref "开始异步调用"(reference=w266, "参数"=w260) -> (reference out=w265:refnum<vi>, error out=w264:errorcluster)  [unwired: 12 in]
            n240 = Close Reference(reference=w265, error in (no error)=w264) -> ()  [unwired: 1 out]
          }
        }
      }
    }
    "选项卡控件" <- "周期设置"
  }
  n241 = while {
    tunnel: w11 -> [w310]
    stop <- FALSE stop-if-true
    n242 = event shown="[7] \"副屏显示设置\": 值改变" {
      selector: _ -> [_ _ _ _ _ _ _ _ _ _ _]
      dyn-events: _ -> [_ _ _ _ _ _ _ _ _ _ _]
      timeout: _ -> [_ _ _ _ _ _ _ _ _ _ _]
      tunnel: w310 -> [_ _ _ _ _ _ _ _ _ w364 _]
      event Timeout {
        n243 = event-data() -> ()  [unwired: 1 in, 3 out]
      }
      event "模块启用配置": Value Change {
        n244 = event-data() -> ()  [unwired: 1 in, 6 out]
        n245 = call "模块启用配置框.vi"() -> ()  [unwired: 12 in]
      }
      event "24H周期设置", "运行模式", "多参数", "CODmn", "氨氮", "总磷总氮", "CODCr", "质控启动日期", "空白核查时间", "跨度核查时间", "运行间隔", "周期设置", "流量阈值", "时间阈值": Value Change {
        n246 = event-data() -> ()  [unwired: 1 in, 6 out]
        n247 = flat-sequence {
          frame #0 {
            n248 = local read "氨氮"() -> (w324:bool)
            n249 = local read "运行间隔"() -> (w315:i16)
            n250 = local read "流量阈值"() -> (w312:dbl)
            n251 = local read "总磷总氮"() -> (w322:bool)
            n252 = local read "周期设置"() -> (w314:enum16{"自由设定", "国标协议", "流量设定"})
            n253 = local read "时间阈值"() -> (w313:u16)
            n254 = local read "运行模式"() -> (w325:enum16{"维护模式", "常规模式", "应急模式", "质控模式"})
            n255 = local read "CODmn"() -> (w321:bool)
            n256 = local read "CODCr"() -> (w323:bool)
            n257 = local read "多参数"() -> (w320:bool)
            n258 = local read "空白核查时间"() -> (w317:u16)
            n259 = local read "质控启动日期"() -> (w318:string)
            n260 = local read "24H周期设置"() -> (w319:bool[])
            n261 = local read "跨度核查时间"() -> (w316:u16)
            n262 = global write "系统设置全局变量.vi" "氨氮自动启动设置"(w324) -> ()
            n263 = global write "系统设置全局变量.vi" "运行间隔"(w315) -> ()
            n264 = global write "系统设置全局变量.vi" "流量阈值"(w312) -> ()
            n265 = global write "系统设置全局变量.vi" "CODCr自动启动设置"(w323) -> ()
            n266 = global write "系统设置全局变量.vi" "总磷总氮自动启动设置"(w322) -> ()
            n267 = global write "系统设置全局变量.vi" "周期设置"(w314) -> ()
            n268 = global write "系统设置全局变量.vi" "CODmn自动启动设置"(w321) -> ()
            n269 = global write "系统设置全局变量.vi" "时间阈值"(w313) -> ()
            n270 = global write "系统设置全局变量.vi" "多参数自动启动设置"(w320) -> ()
            n271 = global write "系统设置全局变量.vi" "运行模式"(w325) -> ()
            n272 = global write "系统设置全局变量.vi" "空白核查时间"(w317) -> ()
            n273 = global write "系统设置全局变量.vi" "质控启动日期"(w318) -> ()
            n274 = global write "系统设置全局变量.vi" "24H周期设置"(w319) -> ()
            n275 = global write "系统设置全局变量.vi" "跨度核查时间"(w316) -> ()
          }
          frame #1 {
            n276 = call <vilib>:"Application Directory.vi"() -> ("Application Directory"=w339:path)
            n277 = Build Path(base path=w339, name or relative path="data\\sys.ini" ("名称或相对路径")) -> (appended path=w337:path)
            n278 = call <vilib>:"Open Config Data.vi"("configuration file path"=w337) -> ("error out"=w333:errorcluster, "refnum"=w336:T1)  [unwired: 8 in, 1 out]
            n279 = vi-ref "系统设置全局变量.vi"() -> (w335:refnum<vi>)
            n280 = call <userlib>:"Write Panel to INI__ogtk.vi"("error in (no error)"=w333, "VI ref"=w335, "refnum"=w336) -> ("error out"=w332:errorcluster, "refnum out"=w334:T1)  [unwired: 7 in]
            n281 = call <vilib>:"Close Config Data.vi"("error in (no error)"=w332, "refnum"=w334) -> ("error out"=w327:errorcluster, "file path"=w326:path)  [unwired: 8 in]
            n282 = Open/Create/Replace File(file path (use dialog)=w326, error in=w327) -> (refnum out=w330:refnum<file>, error out=w331:errorcluster)  [unwired: 4 in, 1 out]
            n283 = Flush File(refnum=w330, error in=w331) -> (refnum out=w329:refnum<file>, error out=w328:errorcluster)
            n284 = Close File(refnum=w329, error in=w328) -> ()  [unwired: 2 out]
          }
        }
      }
      event "运行间隔": Mouse Down {
        n285 = event-data() -> ("CtlRef"=w343:refnum<vi>)  [unwired: 1 in, 7 out]
        n286 = property class="DigNum (严格)"(reference=w343) -> (reference out=w342:refnum<vi>, "Value"=w341:i16)  [unwired: 1 in, 1 out]
        n287 = call "数字键盘.vi"("OldNumber"=w341) -> ("NewNumber"=w340:sgl)
        n288 = property class="DigNum (严格)"(reference=w342, "Val(Sgnl)"=w340) -> ()  [unwired: 1 in, 2 out]
      }
      event "流量阈值": Mouse Down {
        n289 = event-data() -> ("CtlRef"=w347:refnum<vi>)  [unwired: 1 in, 7 out]
        n290 = property class="DigNum (严格)"(reference=w347) -> (reference out=w346:refnum<vi>, "Value"=w345:dbl)  [unwired: 1 in, 1 out]
        n291 = call "数字键盘.vi"("OldNumber"=w345) -> ("NewNumber"=w344:sgl)
        n292 = property class="DigNum (严格)"(reference=w346, "Val(Sgnl)"=w344) -> ()  [unwired: 1 in, 2 out]
      }
      event "时间阈值": Mouse Down {
        n293 = event-data() -> ("CtlRef"=w351:refnum<vi>)  [unwired: 1 in, 7 out]
        n294 = property class="DigNum (严格)"(reference=w351) -> (reference out=w350:refnum<vi>, "Value"=w349:u16)  [unwired: 1 in, 1 out]
        n295 = call "数字键盘.vi"("OldNumber"=w349) -> ("NewNumber"=w348:sgl)
        n296 = property class="DigNum (严格)"(reference=w350, "Val(Sgnl)"=w348) -> ()  [unwired: 1 in, 2 out]
      }
      event "开机启动": Value Change {
        n297 = event-data() -> ("NewVal"=w353:bool)  [unwired: 1 in, 5 out]
        n298 = call <vilib>:"Application Directory.vi"() -> ("Application Directory"=w352:path)
        n299 = case shown="真" w353 {
          tunnel: w352 -> [w355 w359]
          frame False {
            n300 = call "删除启动项.vi"("启动文件路径"=w355) -> ("删除标记"=w354:bool)  [unwired: 9 in, 1 out]
            n301 = case shown="真" w354 {
              frame False {
                n302 = local write "开机启动"(TRUE ("开机启动")) -> ()
                n303 = One Button Dialog(message="启动项删除失败" ("消息")) -> ()  [unwired: 1 in, 1 out]
              }
              frame True {
              }
            }
          }
          frame True {
            n304 = call "添加启动项.vi"("启动文件路径"=w359) -> ("添加成功标记"=w358:bool)  [unwired: 9 in, 1 out]
            n305 = case shown="真" w358 {
              frame False {
                n306 = local write "开机启动"(FALSE ("开机启动")) -> ()
                n307 = One Button Dialog(message="启动项添加失败" ("消息")) -> ()  [unwired: 1 in, 1 out]
              }
              frame True {
              }
            }
          }
        }
      }
      event "副屏显示设置": Value Change {
        n308 = event-data() -> ()  [unwired: 1 in, 6 out]
        n309 = call "副屏设置.vi"() -> ()  [unwired: 12 in]
      }
      event "首页显示设置": Value Change {
        n310 = event-data() -> ()  [unwired: 1 in, 6 out]
        n311 = call "首页显示设置.vi"() -> ()  [unwired: 12 in]
      }
      event "短信报警设置": Value Change {
        n312 = event-data() -> ()  [unwired: 1 in, 6 out]
        n313 = invoke class="VI" method="FP.Open"(reference=w364, "Activate"=TRUE ("激活？"), "State"=T5."Standard" ("状态")) -> ()  [unwired: 2 in, 5 out]
      }
      event "布尔": Value Change {
        n314 = event-data() -> ("OldVal"=w366:bool)  [unwired: 1 in, 5 out]
        n315 = case shown="假" w366 {
          tunnel: [w367 _] -> w365
          frame False {
            n316 = call "数字密码键盘.vi"() -> ("NewNumber"=w367:sgl)  [unwired: 1 in]
          }
          frame True {
          }
        }
        n317 = local write "输入密码"(w365) -> ()
      }
    }
  }
